vi "AlliGator Single SS3 Gate Slip Correction.vi"(8 "error in (no error)":errorcluster, 11 "Refnum in":T1) -> (0 "error out":errorcluster, 1 "Last Strip Saturated?":bool, 3 "Refnum out":T1)   [LabVIEW 2021, in "AlliGator HDF5.lvlib"]
doc: "Removes one of two sets of columns of a SS3 dataset to account for common FPGA data transfer issues."
uses:
  AlliGator HDF5.lvlib
  <vilib>/vision/Image Controls.llb/IMAQ Image.ctl
  SwissSPAD/SwissSPAD Live.lvlib
panel:
  # "see the AlliGator License on the block diagram (Ctrl+E or Window:Show Block Diagram)"
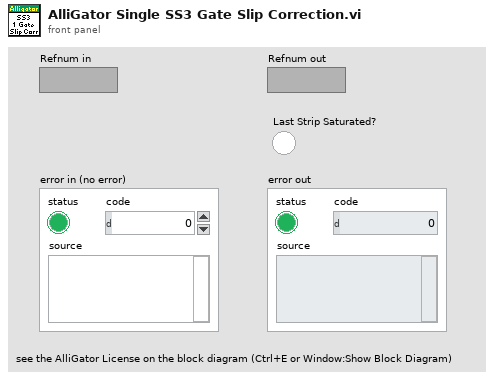
[diagram p1: front panel]
types:
  T1 = typedef "IMAQ Image.ctl" = refnum<image>
  T2 = typedef "Image Type" = u32
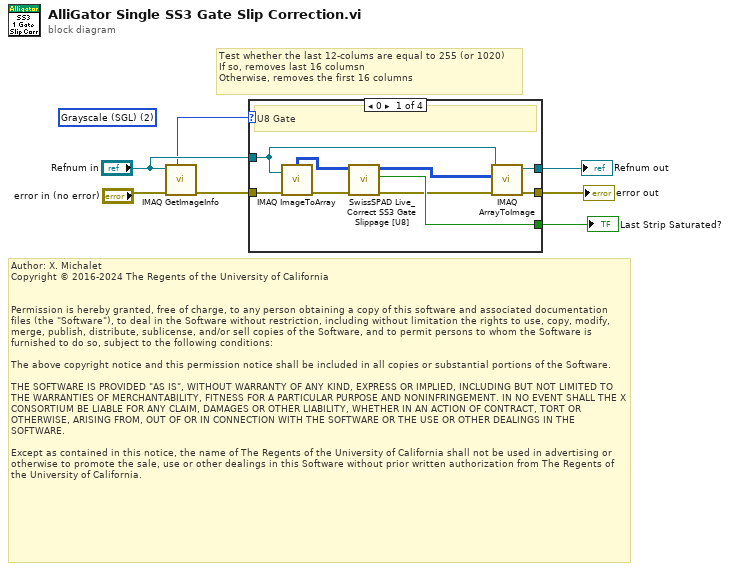
[diagram p0: block diagram]
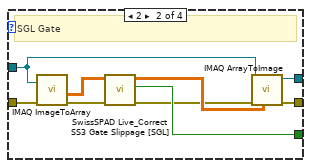
[diagram p2: hidden frame]
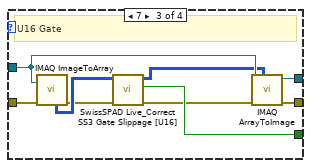
[diagram p3: hidden frame]
diagram:
  (unwired) T2 2 items=["Grayscale (U8)", "Grayscale (I16)", "Grayscale (SGL)", "Complex (CSG)", "RGB (U32)", "HSL (U32)", "RGB (U64)", "Grayscale (U16)"] ("Image Type")
  # "Author: X. Michalet\nCopyright © 2016-2024 The Regents of the University of California\n \n\nPermission is hereby granted, free of charge, to any person obtaining a copy of this software and associated documentation files (the \"Software\"), to deal in the Software without restriction, including without limitation the rights to use, copy, modify, merge, publish, distribute, sublicense, and/or sell copies of the Software, and to permit persons to whom the Software is furnished to do so, subject to the following conditions:\n\nThe above copyright notice and this permission notice shall be included in all copies or substantial portions of the Software.\n\nTHE SOFTWARE IS PROVIDED \"AS IS\", WITHOUT WARRANTY OF ANY KIND, EXPRESS OR IMPLIED, INCLUDING BUT NOT LIMITED TO THE WARRANTIES OF MERCHANTABILITY, FITNESS FOR A PARTICULAR PURPOSE AND NONINFRINGEMENT. IN NO EVENT SHALL THE X CONSORTIUM BE LIABLE FOR ANY CLAIM, DAMAGES OR OTHER LIABILITY, WHETHER IN AN ACTION OF CONTRACT, TORT OR OTHERWISE, ARISING FROM, OUT OF OR IN CONNECTION WITH THE SOFTWARE OR THE USE OR OTHER DEALINGS IN THE SOFTWARE.\n\nExcept as contained in this notice, the name of The Regents of the University of California shall not be used in advertising or otherwise to promote the sale, use or other dealings in this Software without prior written authorization from The Regents of the University of California."
  # "Test whether the last 12-colums are equal to 255 (or 1020)\nIf so, removes last 16 columsn\nOtherwise, removes the first 16 columns"
  n1 = call "IMAQ GetImageInfo"("error in (no error)"="error in (no error)", "Image"="Refnum in") -> ("error out"=w6:errorcluster, "Image Type"=w4:T2)  [unwired: 2 in, 6 out]
  n2 = case shown="0" w4 {
    tunnel: w6 -> [w16 w25 w34 w36]
    tunnel: "Refnum in" -> [w12 w23 w32 w35]
    tunnel: [w13 w24 w33 w36] -> w3
    tunnel: [w11 w22 w31 w35] -> w2
    tunnel: [w10 w19 w28 _] -> w1
    frame 0 {
      # "U8 Gate"
      n3 = call "IMAQ ImageToArray"("error in (no error)"=w16, "Image"=w12) -> ("error out"=w9:errorcluster, "Image Pixels (U8)"=w15:u8[][])  [unwired: 2 in, 3 out]
      n4 = call "SwissSPAD Live_Correct SS3 Gate Slippage [U8].vi"("Error In"=w9, "Array in"=w15) -> ("Error Out"=w8:errorcluster, "Last Strip Saturated?"=w10:bool, "Array out"=w14:u8[][])  [unwired: 7 in]
      n5 = call "IMAQ ArrayToImage"("error in (no error)"=w8, "Image Pixels (U8)"=w14, "Image"=w12) -> ("error out"=w13:errorcluster, "Image Out"=w11:T1)  [unwired: 7 in]
    }
    frame 2 {
      # "SGL Gate"
      n6 = call "IMAQ ImageToArray"("error in (no error)"=w25, "Image"=w23) -> ("Image Pixels (Float)"=w21:sgl[][], "error out"=w18:errorcluster)  [unwired: 2 in, 3 out]
      n7 = call "SwissSPAD Live_Correct SS3 Gate Slippage [SGL].vi"("Error In"=w18, "Array in"=w21) -> ("Error Out"=w17:errorcluster, "Checkbox"=w19:bool, "Array out"=w20:sgl[][])  [unwired: 7 in]
      n8 = call "IMAQ ArrayToImage"("Image Pixels (Float)"=w20, "error in (no error)"=w17, "Image"=w23) -> ("error out"=w24:errorcluster, "Image Out"=w22:T1)  [unwired: 7 in]
    }
    frame 7 {
      # "U16 Gate"
      n9 = call "IMAQ ImageToArray"("error in (no error)"=w34, "Image"=w32) -> ("Image Pixels (U16)"=w30:u16[][], "error out"=w27:errorcluster)  [unwired: 2 in, 3 out]
      n10 = call "SwissSPAD Live_Correct SS3 Gate Slippage [U16].vi"("Error In"=w27, "Array in"=w30) -> ("Error Out"=w26:errorcluster, "Checkbox"=w28:bool, "Array out"=w29:u16[][])  [unwired: 7 in]
      n11 = call "IMAQ ArrayToImage"("Image Pixels (U16)"=w29, "error in (no error)"=w26, "Image"=w32) -> ("error out"=w33:errorcluster, "Image Out"=w31:T1)  [unwired: 7 in]
    }
    frame 1, Default {
      # "not supported"
    }
  }
  "Refnum out" <- w2
  "error out" <- w3
  "Last Strip Saturated?" <- w1
